vi "Launch Actors.vi"(8 "error in (no error)":errorcluster, 10 "Actor":T1(ring), 11 "Main.lvlib:Main.lvclass":refnum<class "Main.lvclass">) -> (0 "error out":errorcluster, 3 "Main.lvlib:Main.lvclass 2":refnum<class "Main.lvclass">)   [LabVIEW 2018, in "Main.lvlib" / "Main.lvclass"]
uses:
  Main.lvclass
  Main.lvclass/Main.ctl
  <vilib>/ActorFramework/Message Enqueuer/Message Enqueuer.lvclass/Message Enqueuer.ctl
  <vilib>/ActorFramework/Message Enqueuer/Enqueue.vi
  <vilib>/ActorFramework/Stop Msg/Stop Msg.lvclass
  C:/Program Files/National Instruments/LabVIEW 2018/vi.lib/ActorFramework/Message/Message.lvclass
  <vilib>/ActorFramework/Message Priority Queue/Priority Enqueue.vi
  MFC Actor/MFC/MFC.lvclass
  Pressure Actor/Pressure/Pressure.lvclass
  Stage Actor/Stage/Stage.lvclass
  Feeder Actor/Feeder/Feeder.lvclass
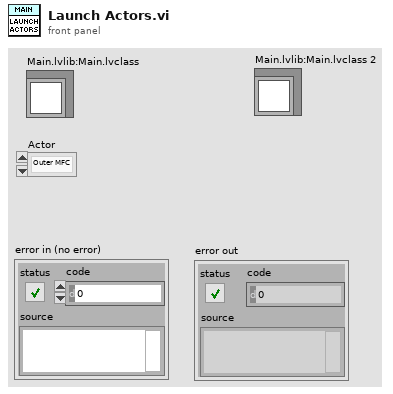
[diagram p1: front panel]
types:
  T1 = enum16{"Outer MFC", "Inner MFC", "Chamber Pressure", "Feeder Pressure", "Stage", "Primary Feeder", "Secondary Feeder", "All"}
  T2 = cluster{"Chamber Pressure":refnum<vi>, "Stage Sub Panel":refnum<vi>, "Feeder Pressure":refnum<vi>, "Inner MFC Sub Panel":refnum<vi>, "Outer MFC Sub Panel":refnum<vi>, "Feeder Sub Panel":refnum<vi>}
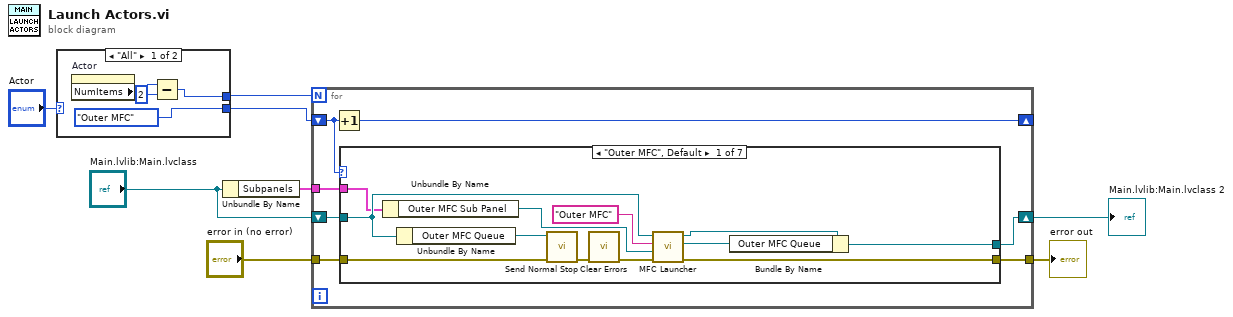
[diagram p0: block diagram]
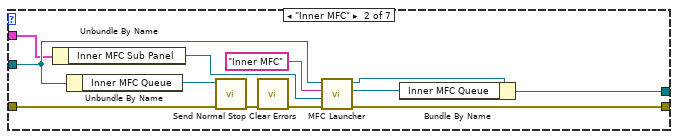
[diagram p2: hidden frame]
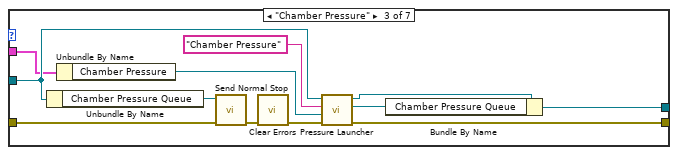
[diagram p3: hidden frame]
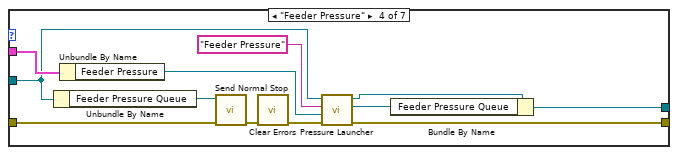
[diagram p4: hidden frame]
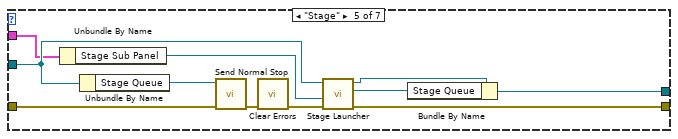
[diagram p5: hidden frame]
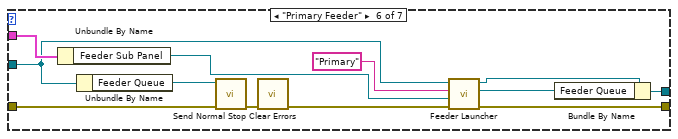
[diagram p6: hidden frame]
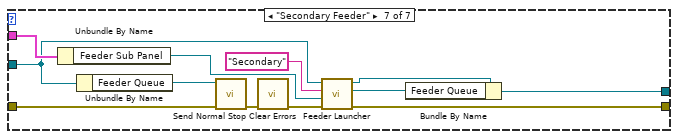
[diagram p7: hidden frame]
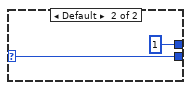
[diagram p8: hidden frame]
diagram:
  n1 = case shown="\"All\"" "Actor" {
    selector: "Actor" -> [_ w13]
    tunnel: [w11 1] -> w5
    tunnel: [T1."Outer MFC" ("Actor") w13] -> w6
    frame "All" {
      n2 = property on="Actor" class="Enum (strict)"() -> ("NumItems"=w10:u32)  [unwired: 2 in, 2 out]
      n3 = Subtract(x=w10, y=u32 2) -> (x-y=w11:u32)
    }
    frame Default {
    }
  }
  n4 = Unbundle By Name("Main.lvlib:Main.lvclass") -> ("Subpanels"=w3:T2)
  n5 = for {
    N: w5 -> [_]
    shift-right: [w21] -> _
    shift-left: w6 -> [w20]
    shift-right: [w15] -> w7
    shift-left: "Main.lvlib:Main.lvclass" -> [w19]
    tunnel: w3 -> [w18]
    tunnel: "error in (no error)" -> [w17]
    tunnel: [w16] -> w1
    n6 = Increment(x=w20) -> (x+1=w21:T1)
    n7 = case shown="\"Outer MFC\", Default" w20 {
      tunnel: w19 -> [w31 w42 w54 w63 w77 w88 w100]
      tunnel: w18 -> [w29 w41 w53 w64 w76 w89 w101]
      tunnel: [w24 w38 w48 w60 w73 w84 w96] -> w15
      tunnel: w17 -> [w26 w36 w51 w66 w79 w82 w95]
      tunnel: [w25 w40 w52 w61 w71 w85 w97] -> w16
      frame "Outer MFC", Default {
        n8 = Unbundle By Name(w29) -> ("Outer MFC Sub Panel"=w33:refnum<vi>)
        n9 = Unbundle By Name(w31) -> ("Outer MFC Queue"=w28:refnum<class "Message Enqueuer.lvclass">)
        n10 = call <vilib>:"Send Normal Stop.vi"("error in (no error)"=w26, "Message Enqueuer"=w28) -> ("error out"=w27:errorcluster)  [unwired: 9 in]
        n11 = call <vilib>:"Clear Errors.vi"("error in (no error)"=w27) -> ("error out"=w22:errorcluster)  [unwired: 5 in, 1 out]
        n12 = call "MFC Launcher.vi"("error in (no error)"=w22, "Sub Panel"=w33, "MFC ID"="Outer MFC", "Panel Actor In"=w31) -> ("error out"=w25:errorcluster, "Nested Actor's Enqueuer"=w23:refnum<class "Message Enqueuer.lvclass">, "Panel Actor Out"=w30:refnum<class "Main.lvclass">)  [unwired: 5 in]
        n13 = Bundle By Name(cluster=w30, "Outer MFC Queue"=w23) -> (w24:refnum<class "Main.lvclass">)
      }
      frame "Inner MFC" {
        n14 = Unbundle By Name(w41) -> ("Inner MFC Sub Panel"=w44:refnum<vi>)
        n15 = Unbundle By Name(w42) -> ("Inner MFC Queue"=w45:refnum<class "Message Enqueuer.lvclass">)
        n16 = call <vilib>:"Send Normal Stop.vi"("error in (no error)"=w36, "Message Enqueuer"=w45) -> ("error out"=w35:errorcluster)  [unwired: 9 in]
        n17 = call <vilib>:"Clear Errors.vi"("error in (no error)"=w35) -> ("error out"=w34:errorcluster)  [unwired: 5 in, 1 out]
        n18 = call "MFC Launcher.vi"("error in (no error)"=w34, "Sub Panel"=w44, "MFC ID"="Inner MFC", "Panel Actor In"=w42) -> ("error out"=w40:errorcluster, "Nested Actor's Enqueuer"=w37:refnum<class "Message Enqueuer.lvclass">, "Panel Actor Out"=w39:refnum<class "Main.lvclass">)  [unwired: 5 in]
        n19 = Bundle By Name(cluster=w39, "Inner MFC Queue"=w37) -> (w38:refnum<class "Main.lvclass">)
      }
      frame "Chamber Pressure" {
        n20 = Unbundle By Name(w54) -> ("Chamber Pressure Queue"=w57:refnum<class "Message Enqueuer.lvclass">)
        n21 = Unbundle By Name(w53) -> ("Chamber Pressure"=w56:refnum<vi>)
        n22 = call <vilib>:"Send Normal Stop.vi"("error in (no error)"=w51, "Message Enqueuer"=w57) -> ("error out"=w50:errorcluster)  [unwired: 9 in]
        n23 = call <vilib>:"Clear Errors.vi"("error in (no error)"=w50) -> ("error out"=w46:errorcluster)  [unwired: 5 in, 1 out]
        n24 = call "Pressure Launcher.vi"("error in (no error)"=w46, "Sub Panel"=w56, "ID"="Chamber Pressure", "Panel Actor In"=w54) -> ("error out"=w52:errorcluster, "Nested Actor's Enqueuer"=w47:refnum<class "Message Enqueuer.lvclass">, "Panel Actor Out"=w49:refnum<class "Main.lvclass">)  [unwired: 5 in]
        n25 = Bundle By Name(cluster=w49, "Chamber Pressure Queue"=w47) -> (w48:refnum<class "Main.lvclass">)
      }
      frame "Feeder Pressure" {
        n26 = Unbundle By Name(w63) -> ("Feeder Pressure Queue"=w69:refnum<class "Message Enqueuer.lvclass">)
        n27 = Unbundle By Name(w64) -> ("Feeder Pressure"=w68:refnum<vi>)
        n28 = call <vilib>:"Send Normal Stop.vi"("error in (no error)"=w66, "Message Enqueuer"=w69) -> ("error out"=w65:errorcluster)  [unwired: 9 in]
        n29 = call <vilib>:"Clear Errors.vi"("error in (no error)"=w65) -> ("error out"=w58:errorcluster)  [unwired: 5 in, 1 out]
        n30 = call "Pressure Launcher.vi"("error in (no error)"=w58, "Sub Panel"=w68, "ID"="Feeder Pressure", "Panel Actor In"=w63) -> ("error out"=w61:errorcluster, "Nested Actor's Enqueuer"=w59:refnum<class "Message Enqueuer.lvclass">, "Panel Actor Out"=w62:refnum<class "Main.lvclass">)  [unwired: 5 in]
        n31 = Bundle By Name(cluster=w62, "Feeder Pressure Queue"=w59) -> (w60:refnum<class "Main.lvclass">)
      }
      frame "Stage" {
        n32 = Unbundle By Name(w76) -> ("Stage Sub Panel"=w78:refnum<vi>)
        n33 = Unbundle By Name(w77) -> ("Stage Queue"=w80:refnum<class "Message Enqueuer.lvclass">)
        n34 = call <vilib>:"Send Normal Stop.vi"("error in (no error)"=w79, "Message Enqueuer"=w80) -> ("error out"=w75:errorcluster)  [unwired: 9 in]
        n35 = call <vilib>:"Clear Errors.vi"("error in (no error)"=w75) -> ("error out"=w70:errorcluster)  [unwired: 5 in, 1 out]
        n36 = call "Stage Launcher.vi"("error in (no error)"=w70, "Sub Panel"=w78, "Panel Actor In"=w77) -> ("error out"=w71:errorcluster, "Nested Actor's Enqueuer"=w72:refnum<class "Message Enqueuer.lvclass">, "Panel Actor Out"=w74:refnum<class "Main.lvclass">)  [unwired: 6 in]
        n37 = Bundle By Name(cluster=w74, "Stage Queue"=w72) -> (w73:refnum<class "Main.lvclass">)
      }
      frame "Primary Feeder" {
        n38 = Unbundle By Name(w89) -> ("Feeder Sub Panel"=w91:refnum<vi>)
        n39 = Unbundle By Name(w88) -> ("Feeder Queue"=w90:refnum<class "Message Enqueuer.lvclass">)
        n40 = call <vilib>:"Send Normal Stop.vi"("error in (no error)"=w82, "Message Enqueuer"=w90) -> ("error out"=w86:errorcluster)  [unwired: 9 in]
        n41 = call <vilib>:"Clear Errors.vi"("error in (no error)"=w86) -> ("error out"=w81:errorcluster)  [unwired: 5 in, 1 out]
        n42 = call "Feeder Launcher.vi"("error in (no error)"=w81, "Sub Panel"=w91, "Feeder ID"="Primary", "Panel Actor In"=w88) -> ("error out"=w85:errorcluster, "Nested Actor's Enqueuer"=w83:refnum<class "Message Enqueuer.lvclass">, "Panel Actor Out"=w87:refnum<class "Main.lvclass">)  [unwired: 5 in]
        n43 = Bundle By Name(cluster=w87, "Feeder Queue"=w83) -> (w84:refnum<class "Main.lvclass">)
      }
      frame "Secondary Feeder" {
        n44 = Unbundle By Name(w101) -> ("Feeder Sub Panel"=w103:refnum<vi>)
        n45 = Unbundle By Name(w100) -> ("Feeder Queue"=w102:refnum<class "Message Enqueuer.lvclass">)
        n46 = call <vilib>:"Send Normal Stop.vi"("error in (no error)"=w95, "Message Enqueuer"=w102) -> ("error out"=w98:errorcluster)  [unwired: 9 in]
        n47 = call <vilib>:"Clear Errors.vi"("error in (no error)"=w98) -> ("error out"=w93:errorcluster)  [unwired: 5 in, 1 out]
        n48 = call "Feeder Launcher.vi"("error in (no error)"=w93, "Sub Panel"=w103, "Feeder ID"="Secondary", "Panel Actor In"=w100) -> ("error out"=w97:errorcluster, "Nested Actor's Enqueuer"=w94:refnum<class "Message Enqueuer.lvclass">, "Panel Actor Out"=w99:refnum<class "Main.lvclass">)  [unwired: 5 in]
        n49 = Bundle By Name(cluster=w99, "Feeder Queue"=w94) -> (w96:refnum<class "Main.lvclass">)
      }
    }
  }
  "error out" <- w1
  "Main.lvlib:Main.lvclass 2" <- w7
